vi "数据查询.vi"() -> ()   [LabVIEW 2016]
uses:
  <vilib>/Utility/miscctls.llb/LVPointTypeDef.ctl
panel:
  in  "数据查询菜单":enum32{"数据查询", "仪器数据", "仪器日志", "报警信息"}(xcontrol)
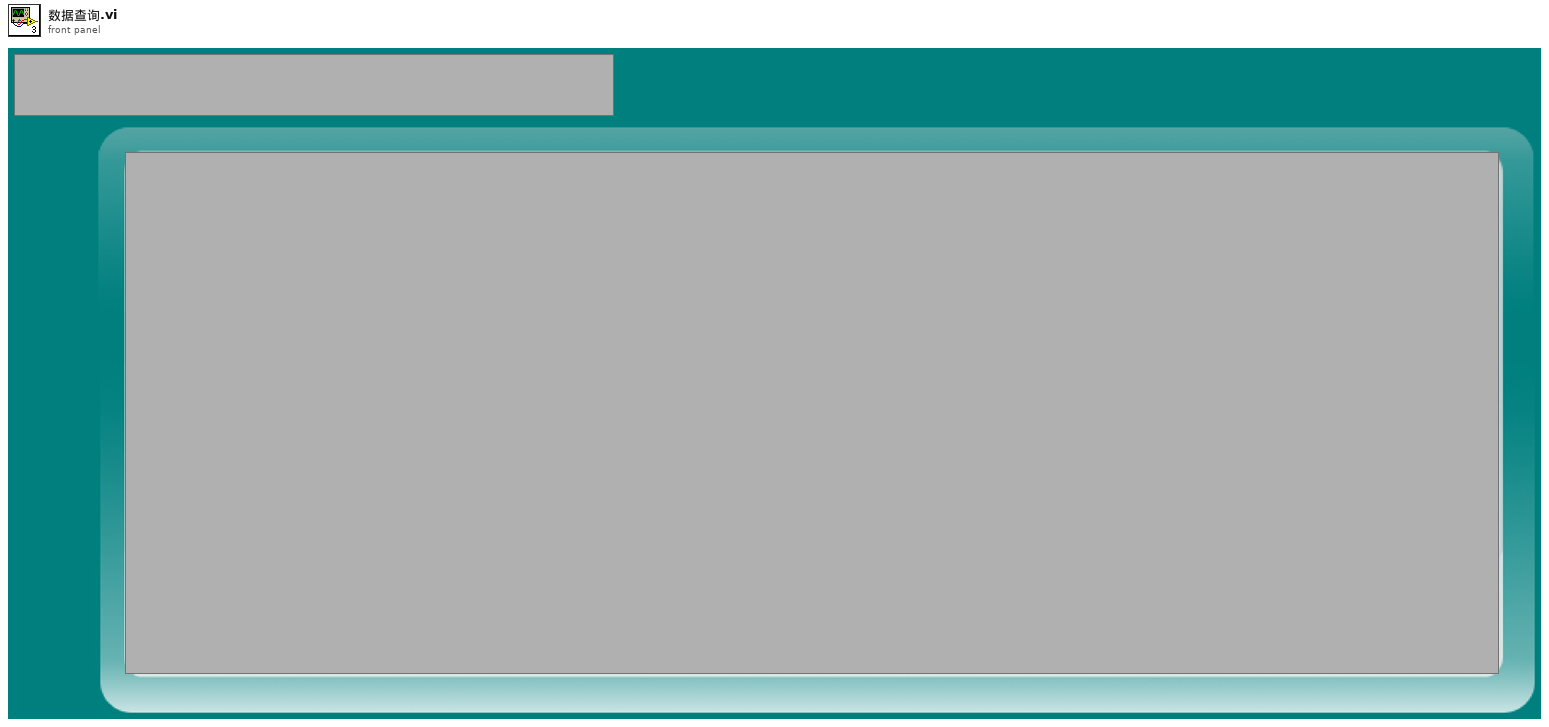
[diagram p1: front panel]
types:
  T1 = typedef "LVPointTypeDef.ctl" = cluster{"Horizontal":i16, "Vertical":i16}
  T2 = enum32{"Bad", "Idle", "Run top level", "Running"}
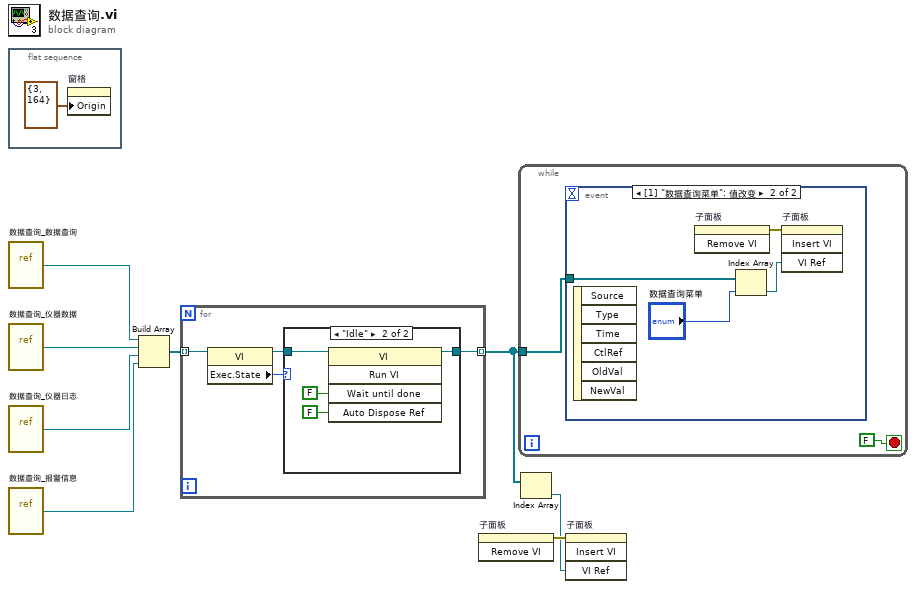
[diagram p0: block diagram]
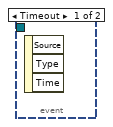
[diagram p3: hidden frame]
diagram:
  n1 = flat-sequence {
    frame #0 {
      n2 = property on="窗格" class="Pane"("Origin"=T1 {"Horizontal"=3, "Vertical"=164} ("原点")) -> ()  [unwired: 2 in, 2 out]
    }
  }
  n3 = vi-ref "数据查询_数据查询.vi"() -> (w5:refnum<vi>)
  n4 = vi-ref "数据查询_仪器数据.vi"() -> (w3:refnum<vi>)
  n5 = vi-ref "数据查询_仪器日志.vi"() -> (w2:refnum<vi>)
  n6 = vi-ref "数据查询_报警信息.vi"() -> (w1:refnum<vi>)
  n7 = Build Array(w5, w3, w2, w1) -> (w4:refnum<vi>[])
  n8 = for {
    tunnel: w4 -> [w13] mode=indexing
    tunnel: [w10] -> w7 mode=indexing
    n9 = property class="VI"(reference=w13) -> (reference out=w11:refnum<vi>, "Exec.State"=w12:T2)  [unwired: 1 in, 1 out]
    n10 = case shown="\"Idle\"" w12 {
      tunnel: w11 -> [w14 w16]
      tunnel: [w14 w15] -> w10
      frame "Bad", Default {
      }
      frame "Idle" {
        n11 = invoke class="VI" method="Run VI"(reference=w16, "Wait until done"=FALSE ("结束前等待"), "Auto Dispose Ref"=FALSE ("自动销毁引用")) -> (reference out=w15:refnum<vi>)  [unwired: 2 in, 4 out]
      }
    }
  }
  n12 = invoke on="子面板" class="SubPnl" method="Remove VI"() -> (error out=w8:errorcluster)  [unwired: 3 in, 2 out]
  n13 = while {
    tunnel: w7 -> [w19]
    stop <- FALSE stop-if-true
    n14 = event shown="[1] \"数据查询菜单\": 值改变" {
      selector: _ -> [_ _]
      dyn-events: _ -> [_ _]
      timeout: _ -> [_ _]
      tunnel: w19 -> [_ w24]
      event Timeout {
        n15 = event-data() -> ()  [unwired: 1 in, 3 out]
      }
      event "数据查询菜单": Value Change {
        n16 = event-data() -> ()  [unwired: 1 in, 6 out]
        n17 = invoke on="子面板" class="SubPnl" method="Remove VI"() -> (error out=w21:errorcluster)  [unwired: 3 in, 2 out]
        n18 = Index Array(array=w24, index="数据查询菜单") -> (element=w22:refnum<vi>)
        n19 = invoke on="子面板" class="SubPnl" method="Insert VI"(error in=w21, "VI Ref"=w22) -> ()  [unwired: 2 in, 4 out]
      }
    }
  }
  n20 = Index Array(array=w7) -> (element=w6:refnum<vi>)  [unwired: 1 in]
  n21 = invoke on="子面板" class="SubPnl" method="Insert VI"(error in=w8, "VI Ref"=w6) -> ()  [unwired: 2 in, 4 out]
